vi "Convert to meters.vi"(8 "error in (no error)":errorcluster, 11 "Lithography Data In":T1(array[cluster])) -> (0 "error out":errorcluster, 3 "Lithography Data Out":T1(array[cluster]))   [LabVIEW 2016]
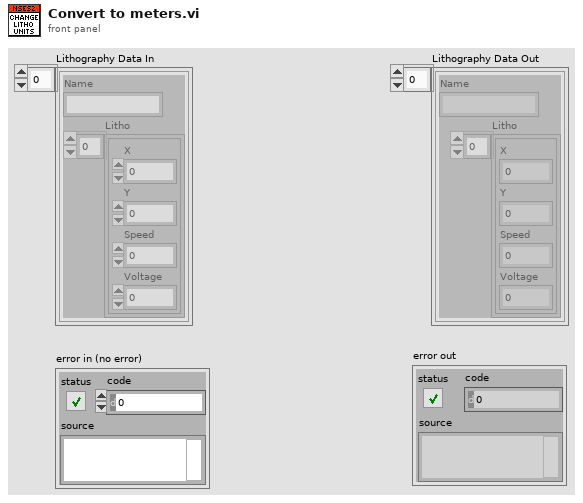
[diagram p1: front panel]
types:
  T1 = cluster{"Name":string, "Litho":cluster{"X":dbl, "Y":dbl, "Speed":dbl, "Voltage":dbl}[]}[]
  T2 = cluster{"X":dbl, "Y":dbl, "Speed":dbl, "Voltage":dbl}[]
  T3 = cluster{"X":dbl, "Y":dbl, "Speed":dbl, "Voltage":dbl}
  T4 = cluster{"Name":string, "Litho":cluster{"X":dbl, "Y":dbl, "Speed":dbl, "Voltage":dbl}[]}
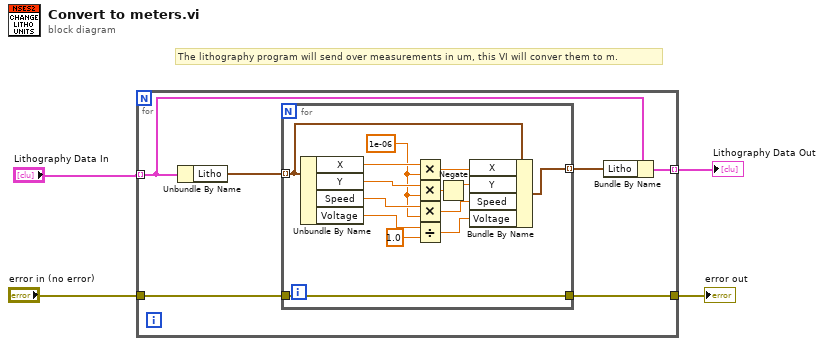
[diagram p0: block diagram]
diagram:
  # "The lithography program will send over measurements in um, this VI will conver them to m."
  n1 = for {
    tunnel: "Lithography Data In" -> [w9] mode=indexing
    tunnel: [w8] -> w4 mode=indexing
    tunnel: "error in (no error)" -> [w6]
    tunnel: [w5] -> w1
    n2 = Unbundle By Name(w9) -> ("Litho"=w10:T2)
    n3 = for {
      tunnel: w10 -> [w20] mode=indexing
      tunnel: [w19] -> w7 mode=indexing
      tunnel: [w11] -> w5
      tunnel: w6 -> [w11]
      w21 = 1e-06 ("y")
      n4 = Unbundle By Name(w20) -> ("X"=w24:dbl, "Y"=w22:dbl, "Speed"=w23:dbl, "Voltage"=w14:dbl)
      n5 = Multiply(x=w24, y=w21) -> (x*y=w18:dbl)
      n6 = Multiply(x=w22, y=w21) -> (x*y=w17:dbl)
      n7 = Multiply(x=w23, y=w21) -> (x*y=w16:dbl)
      n8 = Divide(x=w14, y=1.0) -> (x/y=w12:dbl)
      n9 = Negate(x=w17) -> (-x=w15:dbl)
      n10 = Bundle By Name(cluster=w20, "X"=w18, "Y"=w15, "Speed"=w16, "Voltage"=w12) -> (w19:T3)
    }
    n11 = Bundle By Name(cluster=w9, "Litho"=w7) -> (w8:T4)
  }
  "Lithography Data Out" <- w4
  "error out" <- w1
